vi "Check if Custom Device is Enabled.vi"(8 "error in (no error)":errorcluster, 11 "Ballard ARINC 429 ref":T1 format="%.0x") -> (0 "error out":errorcluster, 2 "Custom Device is Enabled":bool, 3 "Ballard ARINC 429 ref":T1 format="%.0x")   [LabVIEW 2020, in "Ballard ARINC 429 System Explorer.lvlib" / "Implementation.lvlib"]
uses:
  Implementation.lvlib
  <vilib>/NI VeriStand/Custom Device API/Custom Device Item Ref.ctl
  Scripting/Ballard/Ballard ARINC 429 Scripting.lvlib
  <vilib>/NI VeriStand/Custom Device API/Custom Device API.lvlib
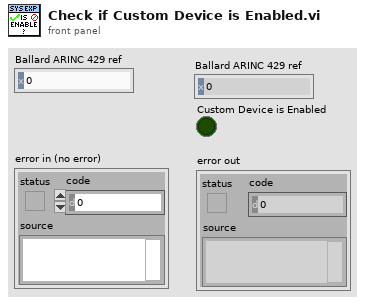
[diagram p1: front panel]
types:
  T1 = typedef "Custom Device API.lvlib/Custom Device Item Ref.ctl" = u64
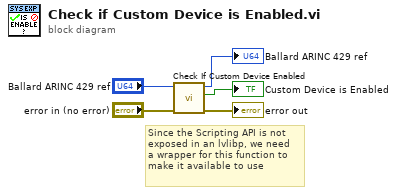
[diagram p0: block diagram]
diagram:
  # "Since the Scripting API is not\nexposed in an lvlibp, we need\na wrapper for this function to\nmake it available to use"
  n1 = call "Check If Custom Device Enabled.vi"("error in (no error)"="error in (no error)", "Ballard ARINC 429 ref"="Ballard ARINC 429 ref") -> ("error out"=→"error out":errorcluster, "Is Custom Device Enabled?"=→"Custom Device is Enabled":bool, "Ballard ARINC 429 ref"=→"Ballard ARINC 429 ref":T1)  [unwired: 7 in]
